vi "CalculateFrames_v03.vi"(8 "Program Spin Coater":T1(array[cluster]), 9 "Seconds End":dbl[unit], 10 "Seconds Start":dbl[unit], 11 "Frame Rate":dbl[unit]) -> (1 "Time":dbl, 2 "Frames":i32)   [LabVIEW 2020]
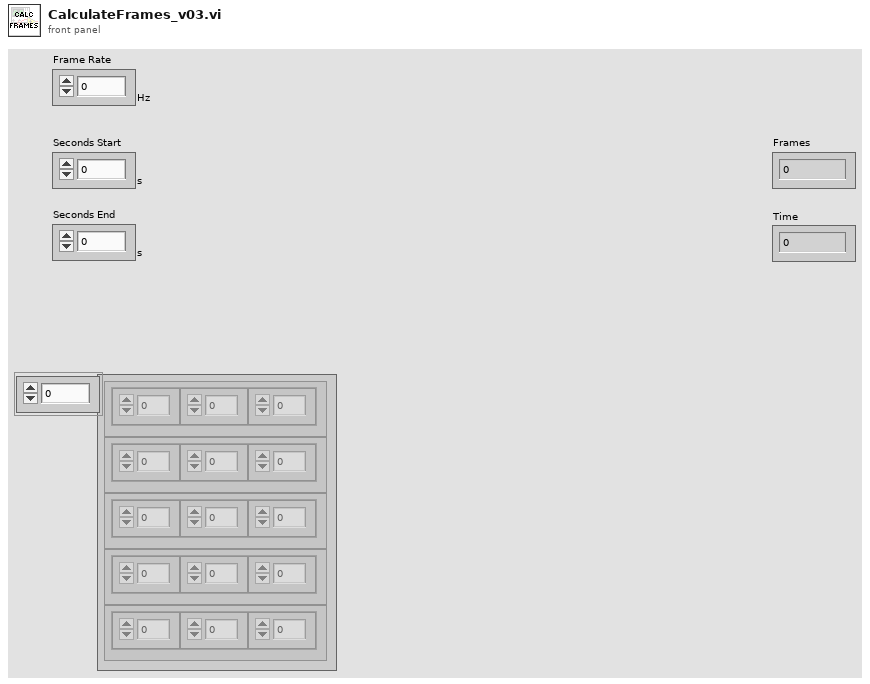
[diagram p1: front panel]
types:
  T1 = cluster{"Speed (rpm)":dbl, "Time (s)":dbl, "Acc (rpm/s)":dbl}[]
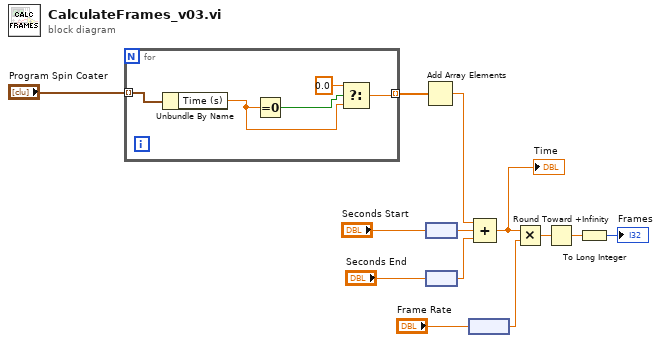
[diagram p0: block diagram]
diagram:
  n1 = for {
    tunnel: "Program Spin Coater" -> [w18] mode=indexing
    tunnel: [w15] -> w1 mode=indexing
    n2 = Unbundle By Name(w18) -> ("Time (s)"=w17:dbl)
    n3 = Equal To 0?(x=w17) -> (x = 0?=w14:bool)
    n4 = Select(t=0.0, s=w14, f=w17) -> (s? t:f=w15:dbl)
  }
  n5 = Add Array Elements(numeric array=w1) -> (sum=w13:dbl)
  n6 = node("Seconds Start") -> (w11:dbl)
  n7 = node("Seconds End") -> (w9:dbl)
  n8 = node("Frame Rate") -> (w6:dbl)
  n9 = Compound Arithmetic op=ADD(w13, w11, w9) -> (w8:dbl)
  "Time" <- w8
  n10 = Multiply(x=w8, y=w6) -> (x*y=w5:dbl)
  n11 = Round Toward +Infinity(x=w5) -> (ceil(x): smallest int >= x=w4:dbl)
  n12 = To Long Integer(number=w4) -> (32bit integer=→"Frames":i32)
